vi "Sagway_Regler.vi"() -> ()   [LabVIEW 2009]
uses:
  <vilib>/NXT/Subs/LVHSConnector.ctl
  <vilib>/NXT/HiTechnic/Sensors/HiTechnic Port.ctl
  <vilib>/NXT/Block Support/NXT_InputPort.ctl
  <vilib>/NXT/Subs/MotorOutput.ctl
  <vilib>/NXT/Block Support/NXT_OutputPort.ctl
  <vilib>/NXT/Dual Mode Library/Waits/Wait_Num.vi
  <vilib>/NXT/Dual Mode Library/Display/drawNumber_float.vi
  <vilib>/NXT/Dual Mode Library/Motors/MotorBrake.vi
  <vilib>/NXT/Dual Mode Library/Waits/Wait_Btn.vi
  <vilib>/NXT/Dual Mode Library/Display/drawText.vi
  <vilib>/NXT/Dual Mode Library/Display/clearDisplay.vi
  <vilib>/NXT/Dual Mode Library/Motors/MotorOn.vi
  <vilib>/NXT/Dual Mode Library/prims/inRangeAndCoerce/inRangeAndCoerce_float.vi
  <vilib>/NXT/Dual Mode Library/Motors/Rotation.vi
  <vilib>/NXT/Dual Mode Library/Sensors/readNXTButton.vi
panel:
  out "NXT":T1={"error"={"status"=FALSE, "code"=0, "source"=""}, "address"="", "NXT #"=-1, "Show Error"=TRUE, "Connection"=4} {"Connection" items=["USB", "Bluetooth", "USB then Bluetooth", "Last Connection", "Preference"]}
  out "t_interval":dbl
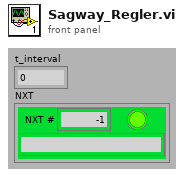
[diagram p1: front panel]
types:
  T1 = typedef "LVHSConnector.ctl" = cluster{"error":errorcluster, "address":string, "NXT #":i32, "Show Error":bool, "Connection":u16}
  T2 = typedef "HiTechnic Port.ctl" = cluster{"Port":T3, "MUX Port":u8}
  T3 = typedef "NXT_InputPort.ctl" = u8
  T4 = typedef "NXT_OutputPort.ctl" = u8
  T5 = typedef "MotorOutput.ctl" = u8
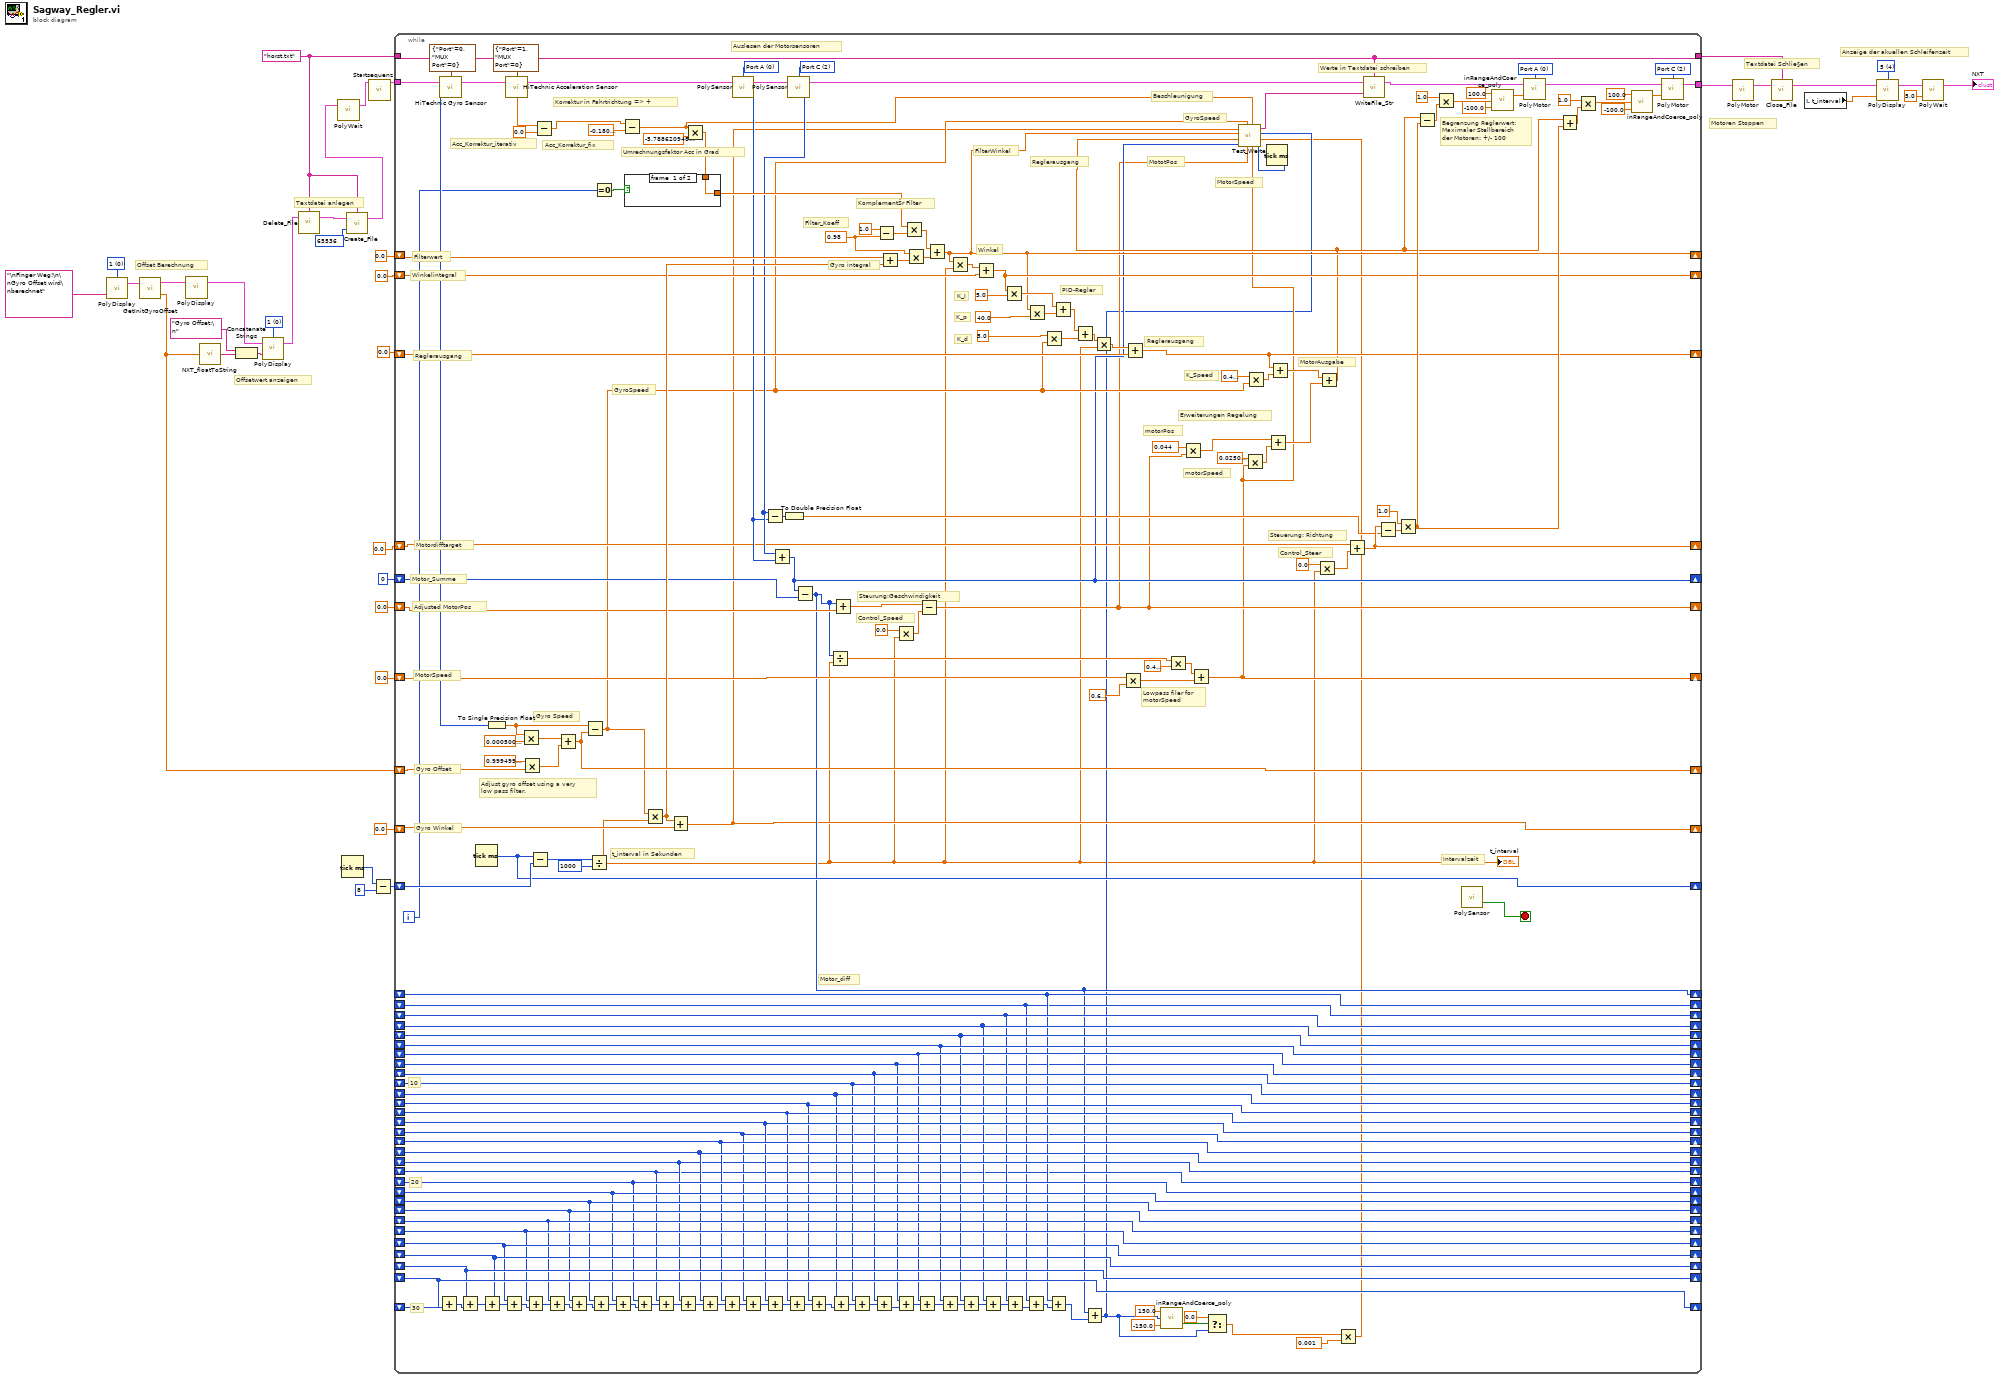
[diagram p0: block diagram]
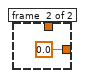
[diagram p2: hidden frame]
diagram:
  w13 = "horst.txt" ("Filename")
  w21 = i16 4 items=["1", "2", "3", "4", "5", "6", "7", "8"] ("Line")
  w29 = i16 0 items=["1", "2", "3", "4", "5", "6", "7", "8"] ("Line")
  w30 = i16 0 items=["1", "2", "3", "4", "5", "6", "7", "8"] ("Line")
  # "Offsetwert anzeigen"
  # "Offset Berechnung"
  # "Textdatei anlegen"
  # "Motoren Stoppen"
  # "Textdatei Schlie§en"
  # "Anzeige der akuellen Schleifenzeit"
  n1 = call-poly <vilib>:"PolyDisplay.vi"("Text"="\nFinger Weg!\n\nGyro Offset wird\nberechnet", "Line"=w30) -> ("NXT"=w32:T1)  [unwired: 2 in]
  n2 = call "GetInitGyroOffset.vi"("NXT"=w32) -> ("GyroOffset"=w23:sgl, "NXT 2"=w28:T1)  [unwired: 1 in]
  n3 = call-poly <vilib>:"PolyDisplay.vi"("NXT"=w28) -> ("NXT"=w24:T1)  [unwired: 3 in]
  n4 = call <vilib>:"NXT_floatToString.vi"("number"=w23) -> ("string"=w26:string)
  n5 = Concatenate Strings("Gyro Offset:\n", w26) -> (w27:string)
  n6 = call-poly <vilib>:"PolyDisplay.vi"("Text"=w27, "NXT"=w24, "Line"=w29) -> ("NXT"=w9:T1)  [unwired: 1 in]
  n7 = call <vilib>:"Delete_File.vi"("NXT"=w9, "Filename"=w13) -> ("NXT"=w14:T1)  [unwired: 2 in]
  n8 = Tick Count (ms)() -> (millisecond timer value=w36:u32)
  n9 = call <vilib>:"Create_File.vi"("File Size (256)"=u32 65536, "NXT"=w14, "Filename"=w13) -> ("NXT"=w7:T1)  [unwired: 1 in]
  n10 = call-poly <vilib>:"PolyWait.vi"("NXT"=w7) -> ("NXT"=w8:T1)  [unwired: 3 in]
  n11 = call "Startsequenz.vi"("NXT"=w8) -> ("NXT 2"=w33:T1)  [unwired: 10 in]
  n12 = Subtract(x=w36, y=u32 8) -> (x-y=w35:u32)
  n13 = while {
    shift-right: [w184] -> _
    shift-left: w35 -> [w215]
    shift-right: [w209] -> _
    shift-left: w23 -> [w208]
    shift-right: [w50] -> _
    shift-left: 0.0 -> [w185]
    tunnel: w33 -> [w206]
    tunnel: [w204] -> w22
    shift-right: [w149] -> _
    shift-left: 0.0 -> [w147]
    shift-right: [w49] -> _
    shift-left: 0.0 -> [w148]
    tunnel: w13 -> [w186]
    tunnel: [w186] -> w10
    shift-right: [w162] -> _
    shift-left: 0.0 -> [w124]
    shift-right: [w156] -> _
    shift-left: 0.0 -> [w157]
    shift-right: [w47] -> _
    shift-left: 0 -> [w140]
    shift-right: [w46] -> _
    shift-left: 0.0 -> [w123]
    shift-right: [w45] -> _
    shift-left: 0.0 -> [w134]
    shift-right: [w63] -> _
    shift-left: _ -> [w68]
    shift-right: [w68] -> _
    shift-left: _ -> [w64]
    shift-right: [w64] -> _
    shift-left: _ -> [w71]
    shift-right: [w71] -> _
    shift-left: _ -> [w73]
    shift-right: [w73] -> _
    shift-left: _ -> [w75]
    shift-right: [w75] -> _
    shift-left: _ -> [w77]
    shift-right: [w77] -> _
    shift-left: _ -> [w79]
    shift-right: [w79] -> _
    shift-left: _ -> [w55]
    shift-right: [w55] -> _
    shift-left: _ -> [w82]
    shift-right: [w82] -> _
    shift-left: _ -> [w84]
    shift-right: [w84] -> _
    shift-left: _ -> [w86]
    shift-right: [w86] -> _
    shift-left: _ -> [w89]
    shift-right: [w89] -> _
    shift-left: _ -> [w91]
    shift-right: [w91] -> _
    shift-left: _ -> [w93]
    shift-right: [w93] -> _
    shift-left: _ -> [w65]
    shift-right: [w65] -> _
    shift-left: _ -> [w96]
    shift-right: [w96] -> _
    shift-left: _ -> [w98]
    shift-right: [w98] -> _
    shift-left: _ -> [w88]
    shift-right: [w88] -> _
    shift-left: _ -> [w66]
    shift-right: [w66] -> _
    shift-left: _ -> [w102]
    shift-right: [w102] -> _
    shift-left: _ -> [w104]
    shift-right: [w104] -> _
    shift-left: _ -> [w106]
    shift-right: [w106] -> _
    shift-left: _ -> [w108]
    shift-right: [w108] -> _
    shift-left: _ -> [w110]
    shift-right: [w110] -> _
    shift-left: _ -> [w112]
    shift-right: [w112] -> _
    shift-left: _ -> [w114]
    shift-right: [w114] -> _
    shift-left: _ -> [w116]
    shift-right: [w116] -> _
    shift-left: _ -> [w118]
    shift-right: [w118] -> _
    shift-left: _ -> [w120]
    shift-right: [w120] -> _
    shift-left: _ -> [w121]
    i -> [w191]
    stop <- w218 stop-if-true
    w169 = T4 2 items=["Port A", "Port B", "Port C"] ("Port (Port A)")
    w170 = T4 0 items=["Port A", "Port B", "Port C"] ("Port (Port A)")
    w174 = T5 2 items=["Port A", "Port B", "Port C", "All Ports"] ("Output Port (All Ports)")
    w175 = T5 0 items=["Port A", "Port B", "Port C", "All Ports"] ("Output Port (All Ports)")
    w199 = 0.98 ("y")
    # "Gyro integral"
    # "Werte in Textdatei schreiben"
    # "Intervalzeit"
    # "Control_Speed"
    # "Steurung:Geschwindigkeit"
    # "Begrenzung Reglerwert:\nMaximaler Stellbereich \nder Motoren: +/- 100"
    # "Auslesen der Motorsensoren"
    # "Erweiterungen Regelung"
    # "Umrechnungsfaktor Acc in Grad"
    # "GyroSpeed"
    # "Beschleunigung"
    # "Acc_Korrektur_iterativ"
    # "Korrektur in Fahrtrichtung => +"
    # "Motor_diff"
    # "30"
    # "20"
    # "10"
    # "MotorSpeed"
    # "MototPos"
    # "GyroSpeed"
    # "Acc_Korrektur_fix"
    # "Winkel"
    # "Reglerausgang"
    # "K_Speed"
    # "motorPos"
    # "motorSpeed"
    # "MotorAusgabe"
    # "MotorSpeed"
    # "Lowpass filer for\nmotorSpeed"
    # "Adjusted MotorPos"
    # "Motor_Summe"
    # "K_I"
    # "Winkelintegral"
    # "Motordifftarget"
    # "Control_Steer"
    # "Steuerung: Richtung"
    # "Filterwert"
    # "Reglerausgang"
    # "FilterWinkel"
    # "Reglerausgang"
    # "PID-Regler"
    # "KomplementŠr Filter"
    # "Filter_Koeff"
    # "t_interval in Sekunden"
    # "K_p"
    # "K_d"
    # "Adjust gyro offset using a very\nlow pass filter."
    # "Gyro Winkel"
    # "Gyro Speed"
    # "Gyro Offset"
    n14 = Add(x=w121, y=w120) -> (x+y=w119:i32)
    n15 = call <vilib>:"HiTechnic Gyro Sensor.vi"("NXT"=w206, "Port/MUX"=T2 {"Port"=0, "MUX Port"=0}) -> ("Gyro Value"=w205:i16, "NXT"=w196:T1)  [unwired: 1 in]
    n16 = Add(x=w118, y=w119) -> (x+y=w117:i32)
    n17 = Tick Count (ms)() -> (millisecond timer value=w184:u32)
    n18 = Add(x=w116, y=w117) -> (x+y=w115:i32)
    n19 = To Single Precision Float(number=w205) -> (single precision float=w210:sgl)
    n20 = Add(x=w114, y=w115) -> (x+y=w113:i32)
    n21 = call <vilib>:"HiTechnic Acceleration Sensor.vi"("NXT"=w196, "Port/MUX"=T2 {"Port"=1, "MUX Port"=0}) -> ("Z Acceleration (m/s^2)"=w57:sgl, "NXT"=w171:T1)  [unwired: 2 in, 2 out]
    n22 = Multiply(x=w210, y=sgl 0.0005) -> (x*y=w212:sgl)
    n23 = Multiply(x=sgl 0.9995 ("y"), y=w208) -> (x*y=w211:sgl)
    n24 = Add(x=w112, y=w113) -> (x+y=w111:i32)
    n25 = Subtract(x=w184, y=w215) -> (x-y=w217:u32)
    n26 = Subtract(x=w57, y=sgl 0.0) -> (x-y=w56:sgl)
    n27 = Add(x=w110, y=w111) -> (x+y=w109:i32)
    n28 = Add(x=w212, y=w211) -> (x+y=w209:sgl)
    n29 = Add(x=w108, y=w109) -> (x+y=w107:i32)
    n30 = Subtract(x=w210, y=w209) -> (x-y=w51:sgl)
    n31 = Divide(x=w217, y=u32 1000) -> (x/y=w38:dbl)
    "t_interval" <- w38
    n32 = Add(x=w106, y=w107) -> (x+y=w105:i32)
    n33 = Equal To 0?(x=w191) -> (x = 0?=w193:bool)
    n34 = Add(x=w104, y=w105) -> (x+y=w103:i32)
    n35 = Subtract(x=w56, y=sgl -0.18) -> (x-y=w41:sgl)
    n36 = Add(x=w102, y=w103) -> (x+y=w101:i32)
    n37 = Multiply(x=w51, y=w38) -> (x*y=w182:dbl)
    n38 = Add(x=w66, y=w101) -> (x+y=w100:i32)
    n39 = Add(x=w182, y=w185) -> (x+y=w50:dbl)
    n40 = Add(x=w88, y=w100) -> (x+y=w99:i32)
    n41 = Multiply(x=w41, y=sgl -5.788621) -> (x*y=w39:sgl)
    n42 = case shown="True" w193 {
      tunnel: [w219 sgl 0.0] -> w183
      tunnel: w39 -> [w219 _]
      frame #0 {
      }
      frame #1 {
      }
    }
    n43 = Add(x=w98, y=w99) -> (x+y=w97:i32)
    n44 = Add(x=w96, y=w97) -> (x+y=w95:i32)
    n45 = call-poly <vilib>:"PolySensor.vi"("NXT"=w171, "Port (Port A)"=w170) -> ("Rotation"=w145:i32, "NXT"=w173:T1)  [unwired: 1 in]
    n46 = Add(x=w65, y=w95) -> (x+y=w94:i32)
    n47 = Add(x=w93, y=w94) -> (x+y=w92:i32)
    n48 = Add(x=w91, y=w92) -> (x+y=w90:i32)
    n49 = call-poly <vilib>:"PolySensor.vi"("NXT"=w173, "Port (Port A)"=w169) -> ("Rotation"=w146:i32, "NXT"=w53:T1)  [unwired: 1 in]
    n50 = Subtract(x=w146, y=w145) -> (x-y=w166:i32)
    n51 = Add(x=w146, y=w145) -> (x+y=w47:i32)
    n52 = To Double Precision Float(number=w166) -> (double precision float=w161:dbl)
    n53 = Subtract(x=w47, y=w140) -> (x-y=w63:i32)
    n54 = Add(x=w89, y=w90) -> (x+y=w87:i32)
    n55 = Divide(x=w63, y=w38) -> (x/y=w135:dbl)
    n56 = Add(x=w86, y=w87) -> (x+y=w85:i32)
    n57 = Add(x=w63, y=w123) -> (x+y=w144:dbl)
    n58 = Add(x=w84, y=w85) -> (x+y=w83:i32)
    n59 = Add(x=w82, y=w83) -> (x+y=w81:i32)
    n60 = Subtract(x=1.0, y=w199) -> (x-y=w197:dbl)
    n61 = Add(x=w148, y=w182) -> (x+y=w187:dbl)
    n62 = Multiply(x=0.0, y=w38) -> (x*y=w143:dbl)
    n63 = Add(x=w55, y=w81) -> (x+y=w80:i32)
    n64 = Multiply(x=w183, y=w197) -> (x*y=w188:dbl)
    n65 = Multiply(x=w199, y=w187) -> (x*y=w198:dbl)
    n66 = Add(x=w79, y=w80) -> (x+y=w78:i32)
    n67 = Subtract(x=w144, y=w143) -> (x-y=w46:dbl)
    n68 = Add(x=w188, y=w198) -> (x+y=w49:dbl)
    n69 = Add(x=w77, y=w78) -> (x+y=w76:i32)
    n70 = Multiply(x=w49, y=w38) -> (x*y=w158:dbl)
    n71 = Add(x=w75, y=w76) -> (x+y=w74:i32)
    n72 = Add(x=w158, y=w157) -> (x+y=w156:dbl)
    n73 = Add(x=w73, y=w74) -> (x+y=w72:i32)
    n74 = Multiply(x=w156, y=5.0) -> (x*y=w154:dbl)
    n75 = Add(x=w71, y=w72) -> (x+y=w70:i32)
    n76 = Add(x=w64, y=w70) -> (x+y=w69:i32)
    n77 = Multiply(x=w49, y=40.0) -> (x*y=w153:dbl)
    n78 = Multiply(x=sgl 5.0, y=w51) -> (x*y=w151:sgl)
    n79 = Add(x=w68, y=w69) -> (x+y=w67:i32)
    n80 = Add(x=w154, y=w153) -> (x+y=w152:dbl)
    n81 = Add(x=w152, y=w151) -> (x+y=w155:dbl)
    n82 = Add(x=w63, y=w67) -> (x+y=w43:i32)
    n83 = Multiply(x=w155, y=w38) -> (x*y=w194:dbl)
    n84 = Multiply(x=w134, y=sgl 0.6) -> (x*y=w139:dbl)
    n85 = Add(x=w194, y=w147) -> (x+y=w149:dbl)
    n86 = call-poly <vilib>:"inRangeAndCoerce_poly.vi"("lower limit"=-150.0, "x"=w43, "upper limit"=150.0) -> ("In Range?"=w60:bool)  [unwired: 1 out]
    n87 = Multiply(x=w135, y=sgl 0.4) -> (x*y=w138:dbl)
    n88 = Multiply(x=0.044, y=w46) -> (x*y=w130:dbl)
    n89 = Add(x=w138, y=w139) -> (x+y=w45:dbl)
    n90 = Select(t=0.0, s=w60, f=w43) -> (s? t:f=w54:dbl)
    n91 = Multiply(x=sgl 0.025, y=w45) -> (x*y=w131:dbl)
    n92 = Multiply(x=sgl 0.4, y=w51) -> (x*y=w150:sgl)
    n93 = Tick Count (ms)() -> (millisecond timer value=w44:u32)
    n94 = Add(x=w130, y=w131) -> (x+y=w129:dbl)
    n95 = Add(x=w149, y=w150) -> (x+y=w141:dbl)
    n96 = Multiply(x=0.0, y=w38) -> (x*y=w165:dbl)
    n97 = Add(x=w141, y=w129) -> (x+y=w48:dbl)
    n98 = Multiply(x=w54, y=0.001) -> (x*y=w42:dbl)
    n99 = call "Test_Werte.vi"("time"=w44, "frei_2"=w42, "frei_1"=w43, "MotorSpeed"=w45, "Beschleunigung"=w41, "MototPos"=w46, "Gyro Speed"=w51, "MotorSumme"=w47, "Reglerausgang"=w48, "FilterWinkel"=w49, "Gyro Winkel"=w50) -> ("concatenated string"=w52:string)
    n100 = Add(x=w124, y=w165) -> (x+y=w162:dbl)
    n101 = call <vilib>:"WriteFile_Str.vi"("String"=w52, "NXT"=w53, "Filename"=w186) -> ("NXT"=w172:T1)  [unwired: 1 in]
    n102 = Subtract(x=w162, y=w161) -> (x-y=w164:dbl)
    n103 = Multiply(x=1.0, y=w164) -> (x*y=w159:dbl)
    n104 = Subtract(x=w48, y=w159) -> (x-y=w168:dbl)
    n105 = Multiply(x=1.0, y=w168) -> (x*y=w178:dbl)
    n106 = call-poly <vilib>:"PolySensor.vi"() -> ("Yes/No"=w218:bool)  [unwired: 3 in, 1 out]
    n107 = call-poly <vilib>:"inRangeAndCoerce_poly.vi"("lower limit"=-100.0, "x"=w178, "upper limit"=100.0) -> ("coerced(x)"=w181:dbl)  [unwired: 1 out]
    n108 = call-poly <vilib>:"PolyMotor.vi"("Power (75)"=w181, "NXT"=w172, "Output Port (All Ports)"=w175) -> ("NXT"=w176:T1)  [unwired: 1 in]
    n109 = Add(x=w48, y=w159) -> (x+y=w167:dbl)
    n110 = Multiply(x=1.0, y=w167) -> (x*y=w190:dbl)
    n111 = call-poly <vilib>:"inRangeAndCoerce_poly.vi"("lower limit"=-100.0, "x"=w190, "upper limit"=100.0) -> ("coerced(x)"=w203:dbl)  [unwired: 1 out]
    n112 = call-poly <vilib>:"PolyMotor.vi"("Power (75)"=w203, "NXT"=w176, "Output Port (All Ports)"=w174) -> ("NXT"=w204:T1)  [unwired: 1 in]
  }
  n113 = call-poly <vilib>:"PolyMotor.vi"("NXT"=w22) -> ("NXT"=w12:T1)  [unwired: 3 in]
  n114 = call <vilib>:"Close_File.vi"("NXT"=w12, "Filename"=w10) -> ("NXT"=w11:T1)  [unwired: 2 in]
  n115 = local read "t_interval"() -> (w15:dbl)
  n116 = call-poly <vilib>:"PolyDisplay.vi"("number"=w15, "NXT"=w11, "Line"=w21) -> ("NXT"=w20:T1)  [unwired: 1 in]
  n117 = call-poly <vilib>:"PolyWait.vi"("Time (1 sec)"=sgl 5.0 ("Time (sec)"), "NXT"=w20) -> ("NXT"=→"NXT":T1)  [unwired: 2 in]
